vi "format write cluster.vi"(10 "type":string, 11 "value":string) -> (2 "Valid ?":bool, 3 "Variant":variant)   [LabVIEW 2020, in "ui-testing.lvlib"]
uses:
  ui-testing.lvlib
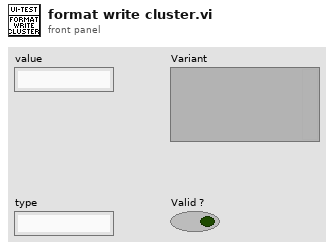
[diagram p1: front panel]
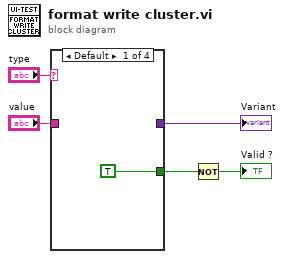
[diagram p0: block diagram]
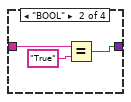
[diagram p2: hidden frame]
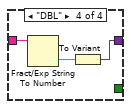
[diagram p4: hidden frame]
diagram:
  n1 = case shown="Default" "type" {
    tunnel: [TRUE _ _ _] -> w3
    tunnel: [_ w7 w10 w13] -> w5
    tunnel: "value" -> [_ w9 w10 w12]
    frame Default {
    }
    frame "BOOL" {
      n2 = Equal?(x=w9, y="True") -> (x = y?=w7:bool)
    }
    frame "STR" {
    }
    frame "DBL" {
      n3 = Fract/Exp String To Number(string=w12) -> (number=w11:dbl)  [unwired: 3 in, 1 out]
      n4 = To Variant(anything=w11) -> (Variant=w13:variant)
    }
  }
  "Variant" <- w5
  n5 = Not(x=w3) -> (.not. x?=→"Valid ?":bool)
